vi "Hamamatsu_Init.vi"(0 "object in":refnum<class "Hamamatsu.lvclass">, 2 "Image Type":T1=7 items=["Grayscale (U8)", "Grayscale (I16)", "Grayscale (SGL)", "Complex (CSG)", "RGB (U32)", "HSL (U32)", "RGB (U64)", "Grayscale (U16)"], 5 "error in (no error)":errorcluster) -> (14 "object out":refnum<class "Hamamatsu.lvclass">, 19 "error out":errorcluster)   [LabVIEW 2019, in "Hamamatsu.lvclass"]
uses:
  Hamamatsu.lvclass
  Hamamatsu.lvclass/Hamamatsu.ctl
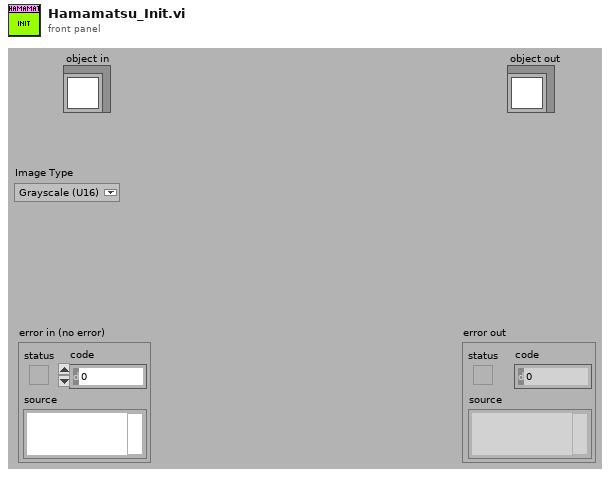
[diagram p1: front panel]
types:
  T1 = typedef "Image Type" = u32
  T2 = cluster{"Capture Library":string, "DCAM-API":string}
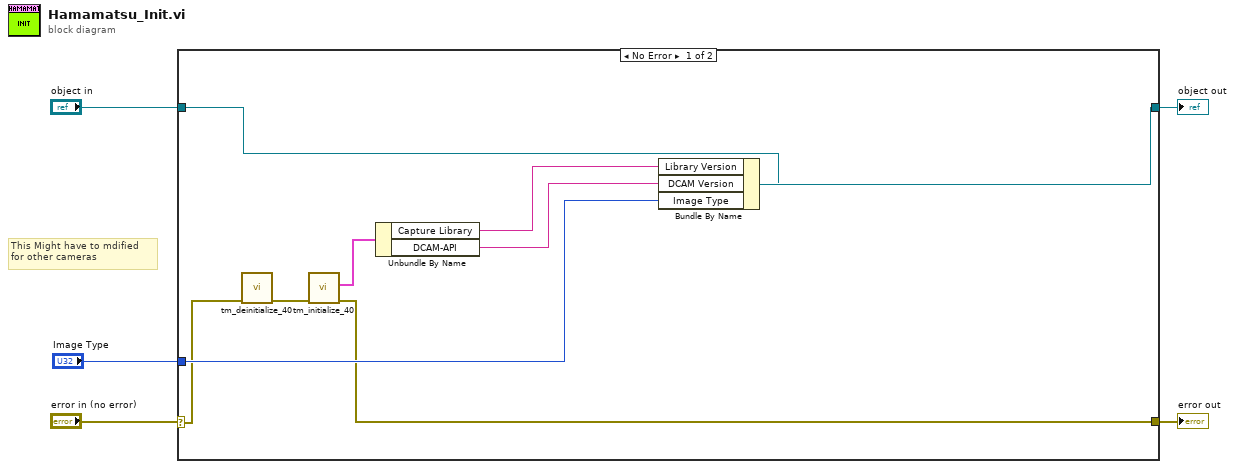
[diagram p0: block diagram]
diagram:
  # "This Might have to mdified \nfor other cameras"
  n1 = case shown="No Error" "error in (no error)" {
    selector: "error in (no error)" -> [w7 w15]
    tunnel: [w14 w16] -> w5
    tunnel: "object in" -> [w13 w16]
    tunnel: [w8 w15] -> w2
    tunnel: "Image Type" -> [w9 _]
    frame No Error {
      n2 = call <userlib>:"tm_deinitialize_40.vi"("error in (no error)"=w7) -> ("error out"=w6:errorcluster)  [unwired: 10 in]
      n3 = call <userlib>:"tm_initialize_40.vi"("error in (no error)"=w6) -> ("error out"=w8:errorcluster, "Version Info"=w12:T2)  [unwired: 7 in, 2 out]
      n4 = Unbundle By Name(w12) -> ("Capture Library"=w11:string, "DCAM-API"=w10:string)
      n5 = Bundle By Name(cluster=w13, "Library Version"=w11, "DCAM Version"=w10, "Image Type"=w9) -> (w14:refnum<class "Hamamatsu.lvclass">)
    }
    frame Error {
    }
  }
  "object out" <- w5
  "error out" <- w2
